vi "NISE.remote.Close Session.vi"(0 "SLSC Remote in":refnum<class "SLSC Interface.lvclass">, 11 "error in (no error)":errorcluster) -> (15 "error out":errorcluster)   [LabVIEW 2016, in "SLSC Interface.lvclass"]
uses:
  SLSC Interface Class/SLSC Interface.lvclass
  SLSC Interface Class/SLSC Interface.lvclass/SLSC Interface.ctl
  SLSC Interface Class/NISE.Read client handle.vi
  SLSC Interface Class/NISE.Read URL.vi
  SLSC Interface Class/NISE.Read session.vi
  <vilib>/httpClient/POSTBuffer.vi
  <vilib>/httpClient/LabVIEWHTTPClient.lvlib
  <vilib>/NI/JSON Support for LabVIEW/JSON Value/JSON Value.lvclass
  <vilib>/NI/NI JSONRPC Server Framework/Classes/Client/JSONRPC Client.lvclass
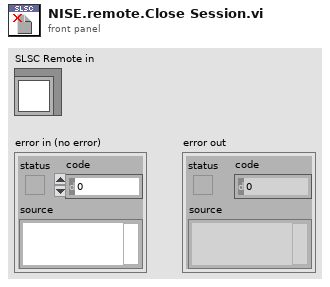
[diagram p1: front panel]
types:
  T1 = typedef "LabVIEWHTTPClient.lvlib/ClientHandle.ctl" = refnum<k1>
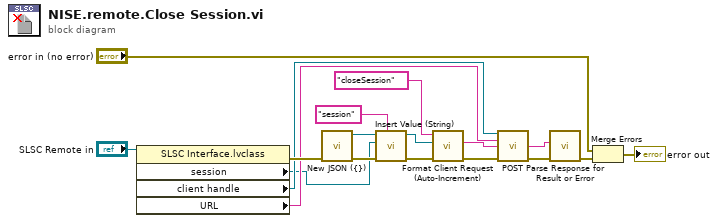
[diagram p0: block diagram]
diagram:
  n1 = property class="SLSC Interface.lvclass"(reference="SLSC Remote in") -> (error out=w17:errorcluster, "session"=w3:refnum<k21>, "client handle"=w11:T1, "URL"=w10:string)  [unwired: 1 in, 1 out]
  n2 = call <vilib>:"New JSON ({}).vi"("error in (no error)"=w17) -> ("error out"=w16:errorcluster, "JSON Value out"=w1:refnum<class "JSON Value.lvclass">)  [unwired: 9 in]
  n3 = call <vilib>:"Insert Value (String).vi"("key"="session" ("Name"), "error in (no error)"=w16, "value"=w3, "JSON Value in"=w1) -> ("error out"=w12:errorcluster, "JSON Value out"=w13:refnum<class "JSON Value.lvclass">)  [unwired: 5 in, 1 out]
  n4 = call <vilib>:"Format Client Request (Auto-Increment).vi"("error in (no error)"=w12, "JSON Value in"=w13, "method"="closeSession") -> ("error out"=w9:errorcluster, "Request String"=w14:string)  [unwired: 7 in]
  n5 = call-poly <vilib>:"POST.vi"("client handle"=w11, "url"=w10, "buffer"=w14, "error in (no error)"=w9) -> ("body"=w8:string, "error out"=w7:errorcluster)  [unwired: 8 in, 2 out]
  n6 = call <vilib>:"Parse Response for Result or Error.vi"("error in"=w7, "Response String In"=w8) -> ("error out"=w6:errorcluster)  [unwired: 7 in, 2 out]
  n7 = Merge Errors("error in (no error)", w6) -> (→"error out":errorcluster)
